vi "Exercise 10.4_Answer.vi"() -> ()   [LabVIEW 2010]
panel:
  in  "stop":bool
  out "Locked/Unlocked":bool
  in  "Clear":bool
  out "Code Entered":string
  in  "Enter":bool
  in  "Button 9":bool
  in  "Button 8":bool
  in  "Button 7":bool
  in  "Button 6":bool
  in  "Button 5":bool
  in  "Button 4":bool
  in  "Button 3":bool
  in  "Button 2":bool
  in  "Button 1":bool
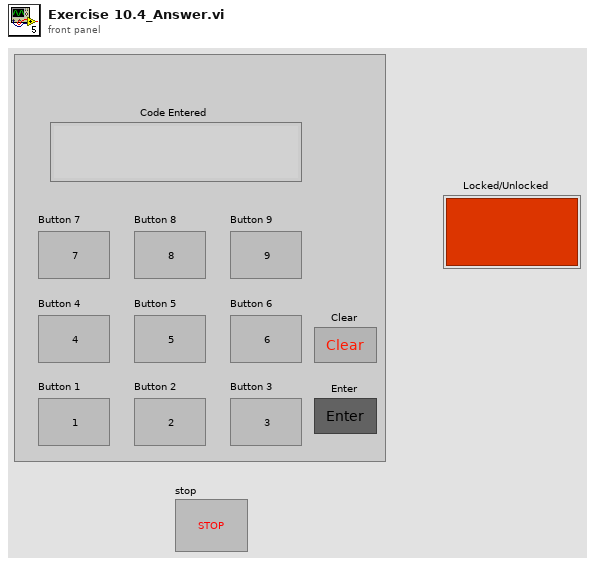
[diagram p1: front panel]
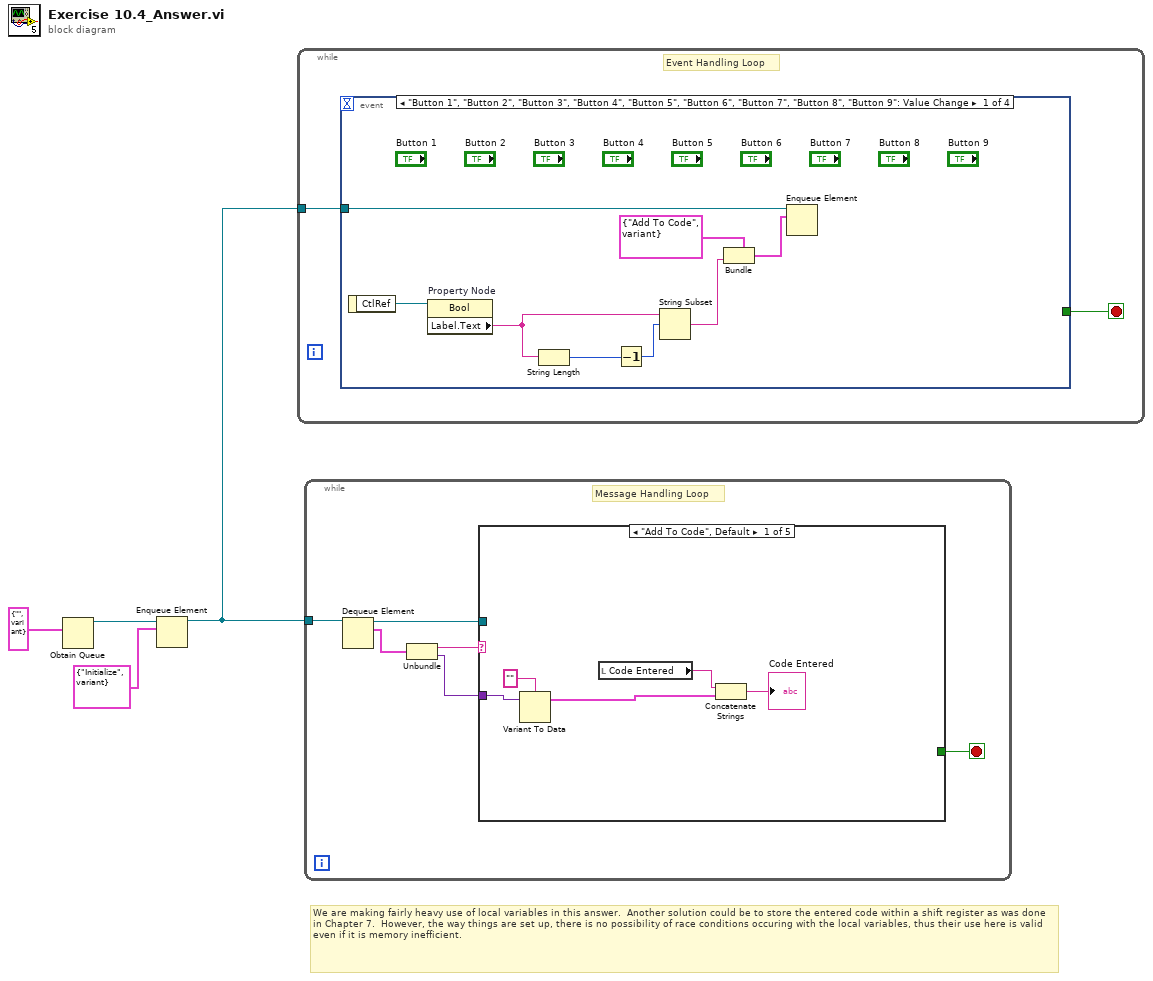
[diagram p0: block diagram]
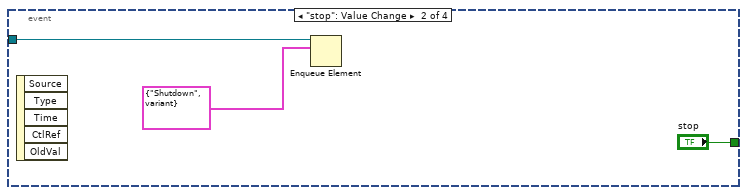
[diagram p2: hidden frame]
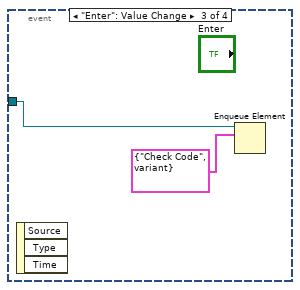
[diagram p3: hidden frame]
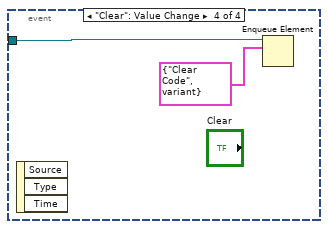
[diagram p4: hidden frame]
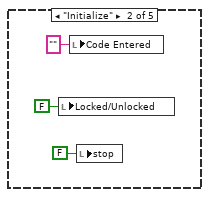
[diagram p5: hidden frame]
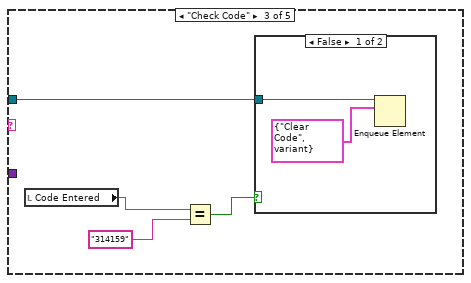
[diagram p6: hidden frame]
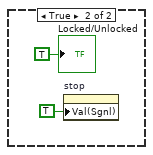
[diagram p7: hidden frame]
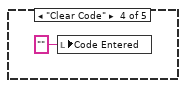
[diagram p8: hidden frame]
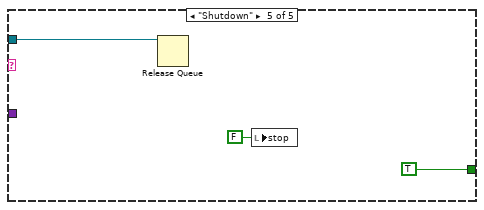
[diagram p9: hidden frame]
diagram:
  # "We are making fairly heavy use of local variables in this answer.  Another solution could be to store the entered code within a shift register as was done in Chapter 7.  However, the way things are set up, there is no possibility of race conditions occuring with the local variables, thus their use here is valid even if it is memory inefficient."
  n1 = Obtain Queue(element data type=cluster{string, variant} {"", variant}) -> (queue out=w3:refnum<queue>)  [unwired: 4 in, 2 out]
  n2 = Enqueue Element(queue=w3, element=cluster{string, variant} {"Initialize", variant}) -> (queue out=w1:refnum<queue>)  [unwired: 2 in, 2 out]
  n3 = while {
    tunnel: w1 -> [w6]
    stop <- w5 stop-if-true
    # "Event Handling Loop"
    n4 = event shown="[0] \"Button 1\", \"Button 2\", \"Button 3\", \"Button 4\", \"Button 5\", \"Button 6\", \"Button 7\", \"Button 8\", \"Button 9\": Value Change" {
      selector: _ -> [_ _ _ _]
      dyn-events: _ -> [_ _ _ _]
      timeout: _ -> [_ _ _ _]
      tunnel: w6 -> [w10 w15 w18 w20]
      tunnel: [_ "stop" _ _] -> w5
      event "Button 1", "Button 2", "Button 3", "Button 4", "Button 5", "Button 6", "Button 7", "Button 8", "Button 9": Value Change {
        n5 = event-data() -> ("CtlRef"=w11:refnum<vi>)  [unwired: 1 in]
        n6 = property on="Property Node" class="Bool"(reference=w11) -> ("Label.Text"=w12:string)  [unwired: 1 in, 2 out]
        n7 = String Length(string=w12) -> (length=w14:i32)
        n8 = Decrement(x=w14) -> (x-1=w13:i32)
        n9 = String Subset(string=w12, offset (0)=w13) -> (substring=w8:string)  [unwired: 1 in]
        n10 = Bundle(cluster=cluster{string, variant} {"Add To Code", variant} ("element"), w8) -> (w7:cluster{string, variant})  [unwired: 1 in]
        n11 = Enqueue Element(queue=w10, element=w7) -> ()  [unwired: 2 in, 3 out]
      }
      event "stop": Value Change {
        n12 = event-data() -> ()  [unwired: 1 in, 5 out]
        n13 = Enqueue Element(queue=w15, element=cluster{string, variant} {"Shutdown", variant}) -> ()  [unwired: 2 in, 3 out]
      }
      event "Enter": Value Change {
        n14 = event-data() -> ()  [unwired: 1 in, 3 out]
        n15 = Enqueue Element(queue=w18, element=cluster{string, variant} {"Check Code", variant}) -> ()  [unwired: 2 in, 3 out]
      }
      event "Clear": Value Change {
        n16 = event-data() -> ()  [unwired: 1 in, 3 out]
        n17 = Enqueue Element(queue=w20, element=cluster{string, variant} {"Clear Code", variant}) -> ()  [unwired: 2 in, 3 out]
      }
    }
  }
  n18 = while {
    tunnel: w1 -> [w27]
    stop <- w22 stop-if-true
    # "Message Handling Loop"
    n19 = Dequeue Element(queue=w27) -> (queue out=w26:refnum<queue>, element=w25:cluster{string, variant})  [unwired: 2 in, 2 out]
    n20 = Unbundle(w25) -> (w24:string, w23:variant)
    n21 = case shown="\"Add To Code\", Default" w24 {
      tunnel: w26 -> [_ _ w36 _ w47]
      tunnel: w23 -> [w31 _ _ _ _]
      tunnel: [_ _ _ _ TRUE] -> w22
      frame "Add To Code", Default {
        n22 = Variant To Data(Variant=w31, type="") -> (data=w29:cluster{})  [unwired: 1 in, 1 out]
        n23 = local read "Code Entered"() -> (w32:string)
        n24 = Concatenate Strings(w32, w29) -> (→"Code Entered":string)
      }
      frame "Initialize" {
        n25 = local write "Locked/Unlocked"(FALSE ("Locked/Unlocked")) -> ()
        n26 = local write "Code Entered"("" ("Code Entered")) -> ()
        n27 = local write "stop"(FALSE ("stop")) -> ()
      }
      frame "Check Code" {
        n28 = local read "Code Entered"() -> (w39:string)
        n29 = Equal?(x=w39, y="314159") -> (x = y?=w37:bool)
        n30 = case shown="False" w37 {
          tunnel: w36 -> [w40 _]
          frame False {
            n31 = Enqueue Element(queue=w40, element=cluster{string, variant} {"Clear Code", variant}) -> ()  [unwired: 2 in, 3 out]
          }
          frame True {
            n32 = property on="stop" class="Bool (strict)"("Val(Sgnl)"=TRUE ("Value (Signaling)")) -> ()  [unwired: 2 in, 2 out]
            "Locked/Unlocked" <- TRUE ("Locked/Unlocked")
          }
        }
      }
      frame "Clear Code" {
        n33 = local write "Code Entered"("" ("Code Entered")) -> ()
      }
      frame "Shutdown" {
        n34 = Release Queue(queue=w47) -> ()  [unwired: 2 in, 3 out]
        n35 = local write "stop"(FALSE ("stop")) -> ()
      }
    }
  }
